vi "Pfeiffer-RVC300.reset.vi"(0 "i ref in":refnum<vi>, 5 "error in (no error)":errorcluster) -> (14 "i ref out":refnum<vi>, 19 "error out":errorcluster)   [LabVIEW 2014, in "Pfeiffer-RVC300.lvlib"]
doc: "This is the constructor of a class.\n\nLicense Agreement for this software:\n\nCopyright (C)\nGesellschaft für Schwerionenforschung, GSI\nPlanckstr. 1\n64291 Darmstadt\nGermany\n\nContact: D.Beck@gsi.de \n\nThis program is free software; you can redistribute it and/or modify it under the terms of the \nGNU General Public License as published by the Free Software Foundation; either version 2 of \nthe license, or (at your option) any later version.\n\nThis program is distributed in the hope that it will be useful, but WITHOUT ANY WARRANTY; \nwithout even the implied warranty of MERCHANTABILITY or FITNESS FOR A PARTICULAR PURPOSE. See the GNU General License for more details (http://www.gnu.org).\n\nGesellschaft für Schwerionenforschung, GSI\nPlanckstr. 1, 64291 Darmstadt, Germany\nFor all questions and ideas contact: M.Richter@gsi.de, H.Brand@gsi.de or D.Beck@gsi.de.\nLast update: 16-JUN-2004"
uses:
  Pfeiffer-RVC300.lvlib
  CS_Core/CSSystem/CoreDefs/CoreDefs.error_type.ctl
  instr.lib/RVC300/RVC-300.lvlib
  CS_Core/CSSystem/CoreLib/CoreLib.lvlib
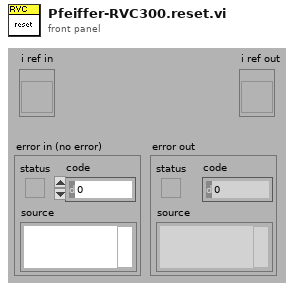
[diagram p1: front panel]
types:
  T1 = typedef "CoreDefs.error_type.ctl" = enum16{"no error", "can't load process", "can't unload process", "process does not exist", "can't install process", "can't remove process", "unknown function", "time out", "can't execute function", "duplicate queue name", "super not found", "caller queue invalid", "can't ping process", "unknown error", "VISA Error", "VISA timeout", "GPIB timeout", "GPIB error", "communication error", "data type mismatch", "can't read data from OPC server", "can't write data to OPC server", "OET error", "function not implemented", "process already exists", "invalid Shared Variable name", "error writing Shared Variable", "error reading Shared Variable", "invalid client name", "corrupt database", "unknown class", "call not authorized", "parameter out of range", "OET timeout: can't get data to modify", "invalid queue name", "requested operation incompatible with current state", "event undefined", "event disabled", "state undefined", "caller is not a friend", "EventBuilder: bad eventID", "EventBuilder: no DAQ devices", "a thread must not stop itself", "UNUSED ELEMENT4", "DiscArchiver: eventData incomplete", "DiscArchiver: eventData does not belong to run", "DiscArchiver: can't open file", "DiscArchiver: can't write to file", "DiscArchiver: available disc space low", "can't acquire semaphore", "error reading data from database", "notifier object is not existing", "can't register process", "can't unregister process", "illegal event type", "object disabled", "object already exists", "can't change state", "Instrument not found", "no connection to remote node", "invalid reference", "N/A", "UNUSED ELEMENT 1", "element not found", "illegal TCP/IP connection detected", "object does not exist", "invalid access ID", "unknown CS system", "invalid privilige", "unsupported data type", "unsupported server type", "IO server already exists", "Shared Variable already exists"}
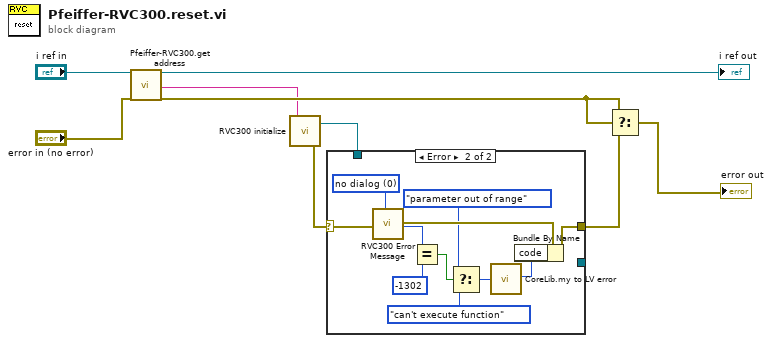
[diagram p0: block diagram]
diagram:
  n1 = call "Pfeiffer-RVC300.get address.vi"("i ref in"="i ref in", "error in (no error)"="error in (no error)") -> ("i ref out"=→"i ref out":refnum<vi>, "address"=w4:string, "error out"=w5:errorcluster)  [unwired: 15 in]
  n2 = call "RVC300 initialize.vi"("RVC300 VISA Resource Name"=w4) -> ("Dup. RVC300 VISA Resource Name"=w1:refnum<visa-resource-name>, "error out"=w3:errorcluster)
  n3 = case shown="Error" w3 {
    selector: w3 -> [w10 w21]
    tunnel: [w10 w18] -> w2
    tunnel: w1 -> [w11 _]
    tunnel: [w11 _] -> _
    frame No Error {
    }
    frame Error {
      w22 = u16 0 items=["no dialog", "OK message", "continue or stop message"] ("type of dialog (OK msg:1)")
      n4 = call "RVC300 Error Message.vi"("error in (no error)"=w21, "type of dialog (OK msg:1)"=w22) -> ("error out"=w20:errorcluster, "code out"=w16:i32)  [unwired: 12 in, 4 out]
      n5 = Equal?(x=w16, y=-1302) -> (x = y?=w17:bool)
      n6 = Select(t=CoreDefs.error_type."parameter out of range" ("ErrorTypes"), s=w17, f=CoreDefs.error_type."can't execute function" ("ErrorTypes")) -> (s? t:f=w12:T1)
      n7 = call "CoreLib.my to LV error.vi"("ErrorTypes"=w12) -> ("LV error code"=w19:i32)  [unwired: 17 in, 1 out]
      n8 = Bundle By Name(cluster=w20, "code"=w19) -> (w18:errorcluster)
    }
  }
  n9 = Select(t=w5, s=w5, f=w2) -> (s? t:f=→"error out":errorcluster)
